vi "_Lock State CSMQ.vi"(8 "Error in":errorcluster caption="Error in (no error)", 11 "CSMQ in":T1) -> (0 "Error out":errorcluster, 2 "lock":bool, 3 "CSMQ out":T1)   [LabVIEW 2014, in "Communicable State Machine.lvlib"]
uses:
  Communicable State Machine.lvlib
  _CSMQ.ctl
  Priority Queue/Priority Queue.lvclass
  Typedef/_CSM_MODE.ctl
  Typedef/_CSM Status Change Event Data.ctl
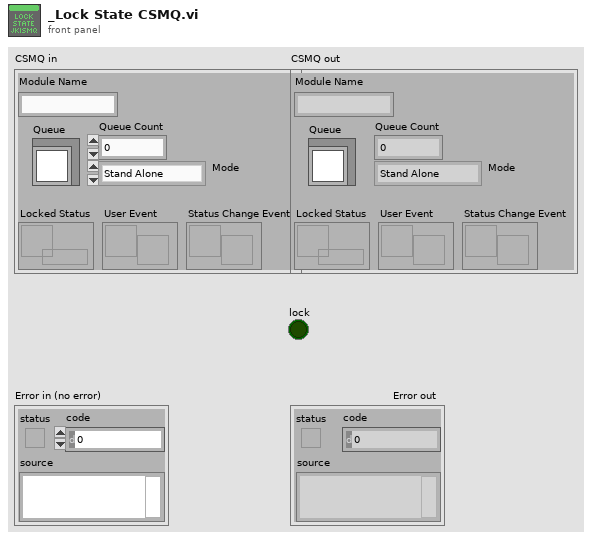
[diagram p1: front panel]
types:
  T1 = typedef "Communicable State Machine.lvlib/_CSMQ.ctl" = cluster{"Module Name":string, "Queue":refnum<class "Priority Queue.lvclass">, "Locked Status":refnum<data-value>, "Mode":T2, "User Event":refnum<user-event>, "Queue Count":i32, "Status Change Event":refnum<user-event>}
  T2 = typedef "Communicable State Machine.lvlib/_CSM_MODE.ctl" = enum16{"Stand Alone", "CSM", "Action Worker"}
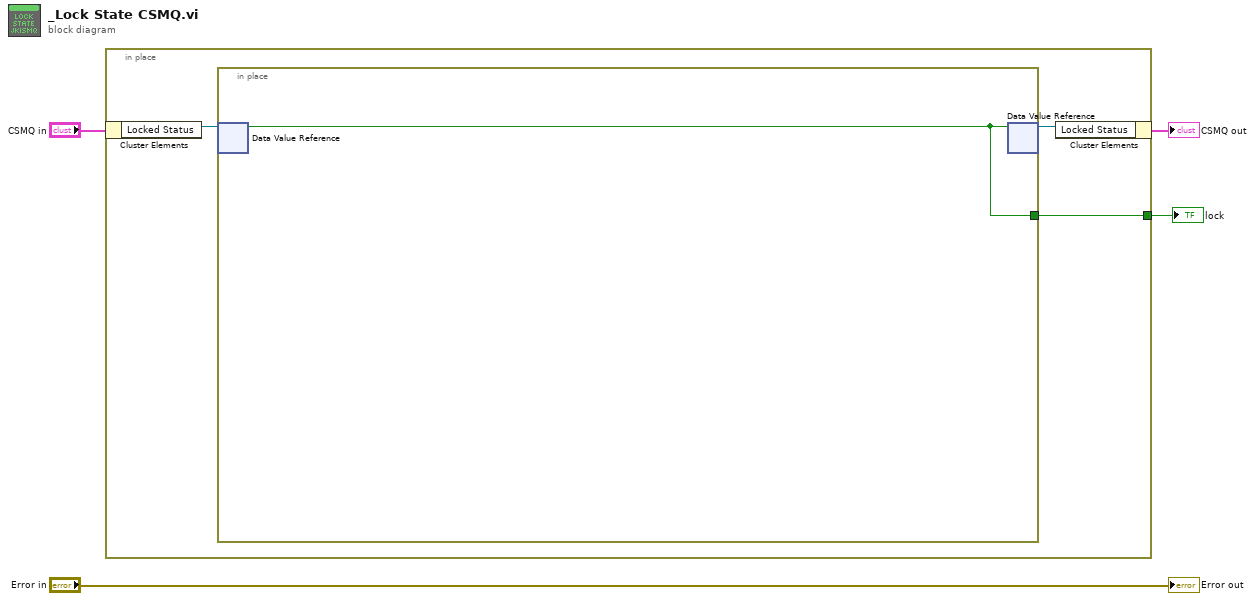
[diagram p0: block diagram]
diagram:
  n1 = in-place "In Place Element Structure" {
    in-place-border: [w5] -> w1
    n2 = in-place-cluster #1("CSMQ in") -> ("Locked Status"=w7:refnum<data-value>)
    n3 = in-place {
      in-place-border: [w8] -> w5
      n4 = in-place-dvr #2(w7) -> (w8:bool)  [unwired: 1 out]
      n5 = in-place-dvr #2(w8) -> (w6:refnum<data-value>)  [unwired: 1 out]
    }
    n6 = in-place-cluster #1("Locked Status"=w6) -> (→"CSMQ out":T1)
  }
  "lock" <- w1
  "Error out" <- "Error in"
